vi "Construct Formatted String Binding.vi"(7 "Format String":string, 10 "Str Refnum":refnum<vi>) -> (0 "error out":errorcluster, 3 "FormattedStringBinding":refnum<class "FormattedStringBinding.lvclass">)   [LabVIEW 2019, in "FormattedStringBinding.lvclass"]
doc: "<License>\nCopyright © 2017 Composed Systems, LLC | All rights reserved\nwww.composed.io\n\nAuthor: Ethan Stern <ethan.stern@composed.io>\n\nThis software is provided \"AS IS\" WITHOUT WARRANTIES, either express or implied, AND IS FOR EDUCATIONAL PURPOSES ONLY.\n</License>"
uses:
  <vilib>/gpm_packages/@cs/transport/Source/Concrete/FormattedStringBinding/FormattedStringBinding.lvclass
  C:/Program Files/National Instruments/LabVIEW 2019/vi.lib/gpm_packages/@cs/transport/Source/Concrete/TerminalValueBinding/TerminalValueBinding.lvclass
  <vilib>/gpm_packages/@cs/transport/Source/Concrete/FormattedStringBinding/FormattedStringBinding.lvclass/FormattedStringBinding.ctl
  <vilib>/Utility/error.llb/Error Cluster From Error Code.vi
  <vilib>/ErrorRing/Error Ring.xnode
  <vilib>/gpm_packages/@cs/transport/Source/Concrete/TerminalValueBinding/TerminalValueBinding.lvclass
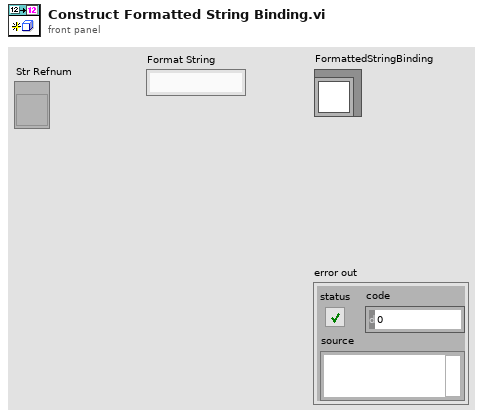
[diagram p1: front panel]
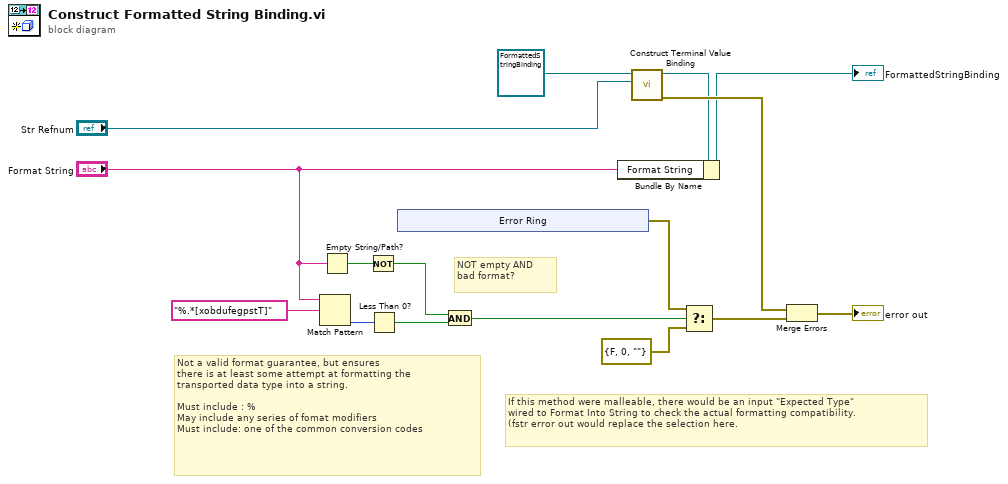
[diagram p0: block diagram]
diagram:
  # "NOT empty AND\nbad format?"
  # "If this method were malleable, there would be an input \"Expected Type\"\nwired to Format Into String to check the actual formatting compatibility.\n(fstr error out would replace the selection here."
  # "Not a valid format guarantee, but ensures\nthere is at least some attempt at formatting the\ntransported data type into a string.\n\nMust include : %\nMay include any series of fomat modifiers\nMust include: one of the common conversion codes"
  n1 = Match Pattern(string="Format String", regular expression="%.*[xobdufegpstT]") -> (offset past match=w10:i32)  [unwired: 1 in, 3 out]
  n2 = Empty String/Path?(string/path="Format String") -> (empty?=w3:bool)
  n3 = Not(x=w3) -> (.not. x?=w1:bool)
  n4 = Less Than 0?(x=w10) -> (x < 0?=w9:bool)
  n5 = xnode "Error Ring"() -> ("error out"=w7:errorcluster)
  n6 = And(x=w1, y=w9) -> (x .and. y?=w2:bool)
  n7 = call <vilib>:"Construct Terminal Value Binding.vi"("Ctl Refnum"="Str Refnum", "TerminalValueBinding In"=refnum<class "FormattedStringBinding.lvclass"> refnum ("FormattedStringBinding.lvclass")) -> ("error out"=w16:errorcluster, "TerminalValueBinding Out"=w13:refnum<class "FormattedStringBinding.lvclass">)  [unwired: 8 in]
  n8 = Bundle By Name(cluster=w13, "Format String"="Format String") -> (→"FormattedStringBinding":refnum<class "FormattedStringBinding.lvclass">)
  n9 = Select(t=w7, s=w2, f=errorcluster {"status"=FALSE, "code"=0, "source"=""} ("error constant")) -> (s? t:f=w5:errorcluster)
  n10 = Merge Errors(w16, w5) -> (→"error out":errorcluster)
